vi "setParameters.vi"(0 "Interface in":T2, 5 "Parameters":T1, 11 "error in":errorcluster) -> (4 "Interface out":T2, 15 "error out":errorcluster)   [LabVIEW 2017, in "AFE_interface.lvlib"]
uses:
  AFE_interface.lvlib
  InterfaceRef.ctl
  <instrlib>/_niInstr/Instruction Framework/v1/Host/Instruction Target/niInstr Instruction Target v1 Host.lvclass
  <instrlib>/_niInstr/Instruction Framework/v1/Host/Instruction Framework Context/niInstr Instruction Framework Context v1 Host.lvclass
  AFE/Parameters.ctl
  AFE/ActiveFrontEnd.lvlib
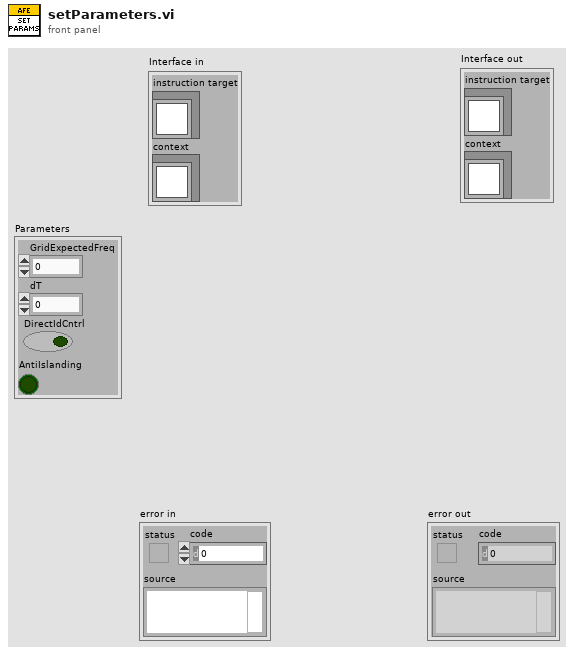
[diagram p1: front panel]
types:
  T1 = typedef "ActiveFrontEnd.lvlib/Parameters.ctl" = cluster{"GridExpectedFreq":sgl, "dT":sgl, "DirectIdCntrl":bool, "AntiIslanding":bool}
  T2 = typedef "AFE_interface.lvlib/InterfaceRef.ctl" = cluster{"instruction target":refnum<class "niInstr Instruction Target v1 Host.lvclass">, "context":refnum<class "niInstr Instruction Framework Context v1 Host.lvclass">}
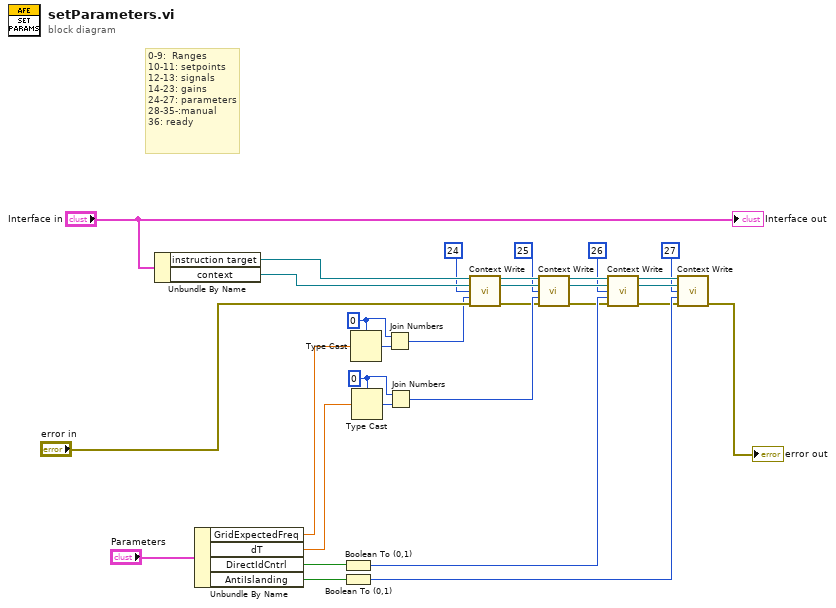
[diagram p0: block diagram]
diagram:
  w21 = u32 0
  w27 = u32 0
  # "0-9:  Ranges\n10-11: setpoints\n12-13: signals\n14-23: gains\n24-27: parameters\n28-35-:manual\n36: ready"
  n1 = Unbundle By Name("Interface in") -> ("instruction target"=w30:refnum<class "niInstr Instruction Target v1 Host.lvclass">, "context"=w29:refnum<class "niInstr Instruction Framework Context v1 Host.lvclass">)
  n2 = Unbundle By Name("Parameters") -> ("GridExpectedFreq"=w23:sgl, "dT"=w20:sgl, "DirectIdCntrl"=w19:bool, "AntiIslanding"=w18:bool)
  n3 = Boolean To (0,1)(Boolean=w19) -> (0, 1=w6:i16)
  n4 = Boolean To (0,1)(Boolean=w18) -> (0, 1=w5:i16)
  n5 = Type Cast(type=w27, x=w23) -> (*(type *) &x=w26:u32)
  n6 = Type Cast(type=w21, x=w20) -> (*(type *) &x=w22:u32)
  n7 = Join Numbers(hi=w27, lo=w26) -> ((hi.lo)=w25:u64)
  n8 = Join Numbers(hi=w21, lo=w22) -> ((hi.lo)=w7:u64)
  n9 = call <instrlib>:"Context Write.vi"("instruction target in"=w30, "context in"=w29, "address"=u64 24, "data"=w25, "error in"="error in") -> ("instruction target out"=w16:refnum<class "niInstr Instruction Target v1 Host.lvclass">, "context out"=w13:refnum<class "niInstr Instruction Framework Context v1 Host.lvclass">, "error out"=w4:errorcluster)  [unwired: 8 in]
  n10 = call <instrlib>:"Context Write.vi"("instruction target in"=w16, "context in"=w13, "address"=u64 25, "data"=w7, "error in"=w4) -> ("instruction target out"=w15:refnum<class "niInstr Instruction Target v1 Host.lvclass">, "context out"=w12:refnum<class "niInstr Instruction Framework Context v1 Host.lvclass">, "error out"=w3:errorcluster)  [unwired: 8 in]
  n11 = call <instrlib>:"Context Write.vi"("instruction target in"=w15, "context in"=w12, "address"=u64 26, "data"=w6, "error in"=w3) -> ("instruction target out"=w14:refnum<class "niInstr Instruction Target v1 Host.lvclass">, "context out"=w11:refnum<class "niInstr Instruction Framework Context v1 Host.lvclass">, "error out"=w2:errorcluster)  [unwired: 8 in]
  n12 = call <instrlib>:"Context Write.vi"("instruction target in"=w14, "context in"=w11, "address"=u64 27, "data"=w5, "error in"=w2) -> ("error out"=→"error out":errorcluster)  [unwired: 8 in, 2 out]
  "Interface out" <- "Interface in"
